vi "AutonGlobal.vi"() -> ()   [LabVIEW 2020]
panel:
  out "Auton On":bool
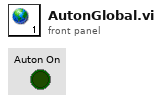
[diagram p1: front panel]
diagram:
